vi "bigcryo_Harry-IcT - v1.vi"() -> ()   [LabVIEW 2019]
uses:
  <vilib>/Utility/file.llb/Read From Spreadsheet File (DBL).vi
panel:
  in  "Settle Time (s)":dbl=60.0
  in  "Step/Ramp":bool=TRUE
  in  "T Rate (K/min)":dbl=0.1
  out "Sample Temp - Idle [K]":dbl=1.997
  in  "LakeShore340":refnum<visa-resource-name>="COM7"
  out "dV/dI-I":cluster{dbl[], dbl[]}(graph) caption="XY Graph"
  out "I-V":cluster{dbl[], dbl[]}(graph) caption="XY Graph"
  out "Status":string="Measuring..."
  in  "Stop":bool
  in  "Keithley":refnum<visa-resource-name>="GPIB1::20::INSTR"
  in  "Delay [sec]":dbl=0.002 format="%#_6e"
  in  "Compliance [V] 2":dbl=10.0 format="%#_6f"
  in  "Delta [A]":dbl=1e-05 format="%#_6e"
  in  "Abort Conductance":bool
  in  "Step [A]":dbl=1e-05 format="%#_6e"
  in  "I-Max [A]":dbl=0.002 format="%#_6e"
  in  "Arm Conductance":bool
  in  "Measure":bool
  in  "Directory Output":string="C:\\User Data\\hlb54\\210111_42B\\JJ1\\IcT_test"
  out "T Now":string="2.010"
  in  "Minicryo":bool=TRUE
  in  "Field and rate":dbl[][](array[numeric])
  in  "step":bool=TRUE
  in  "Magnet VISA?":refnum<visa-resource-name>="COM6"
  out "?":refnum<visa-resource-name>="GPIB1::20::INSTR"
  out "Iteration?":i32=401
  out "Path Out":path=path "C:/User Data/hlb54/gigi.dat"
  in  "Start Temp (K)":dbl=2.0 format="%#_7f"
  in  "T Step (K)":dbl=0.01
  out "T Aim":dbl=2.02
  in  "Stop Temp (K)":dbl=2.1
  # "Step"
  # "Ramp"
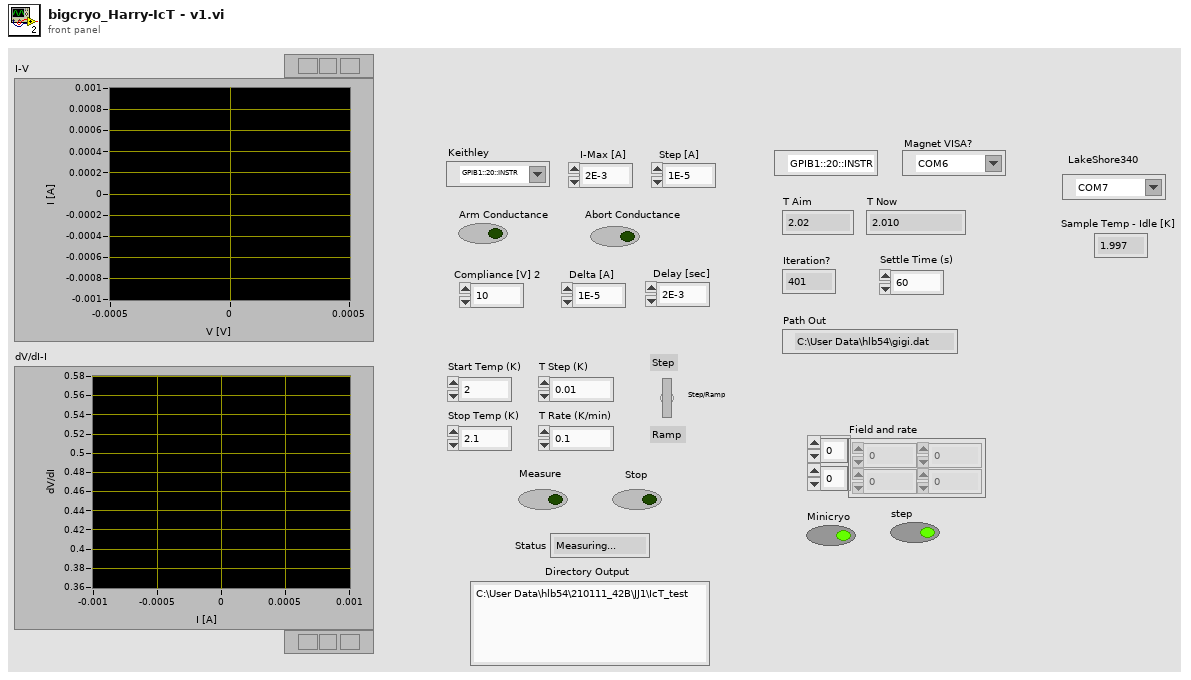
[diagram p1: front panel]
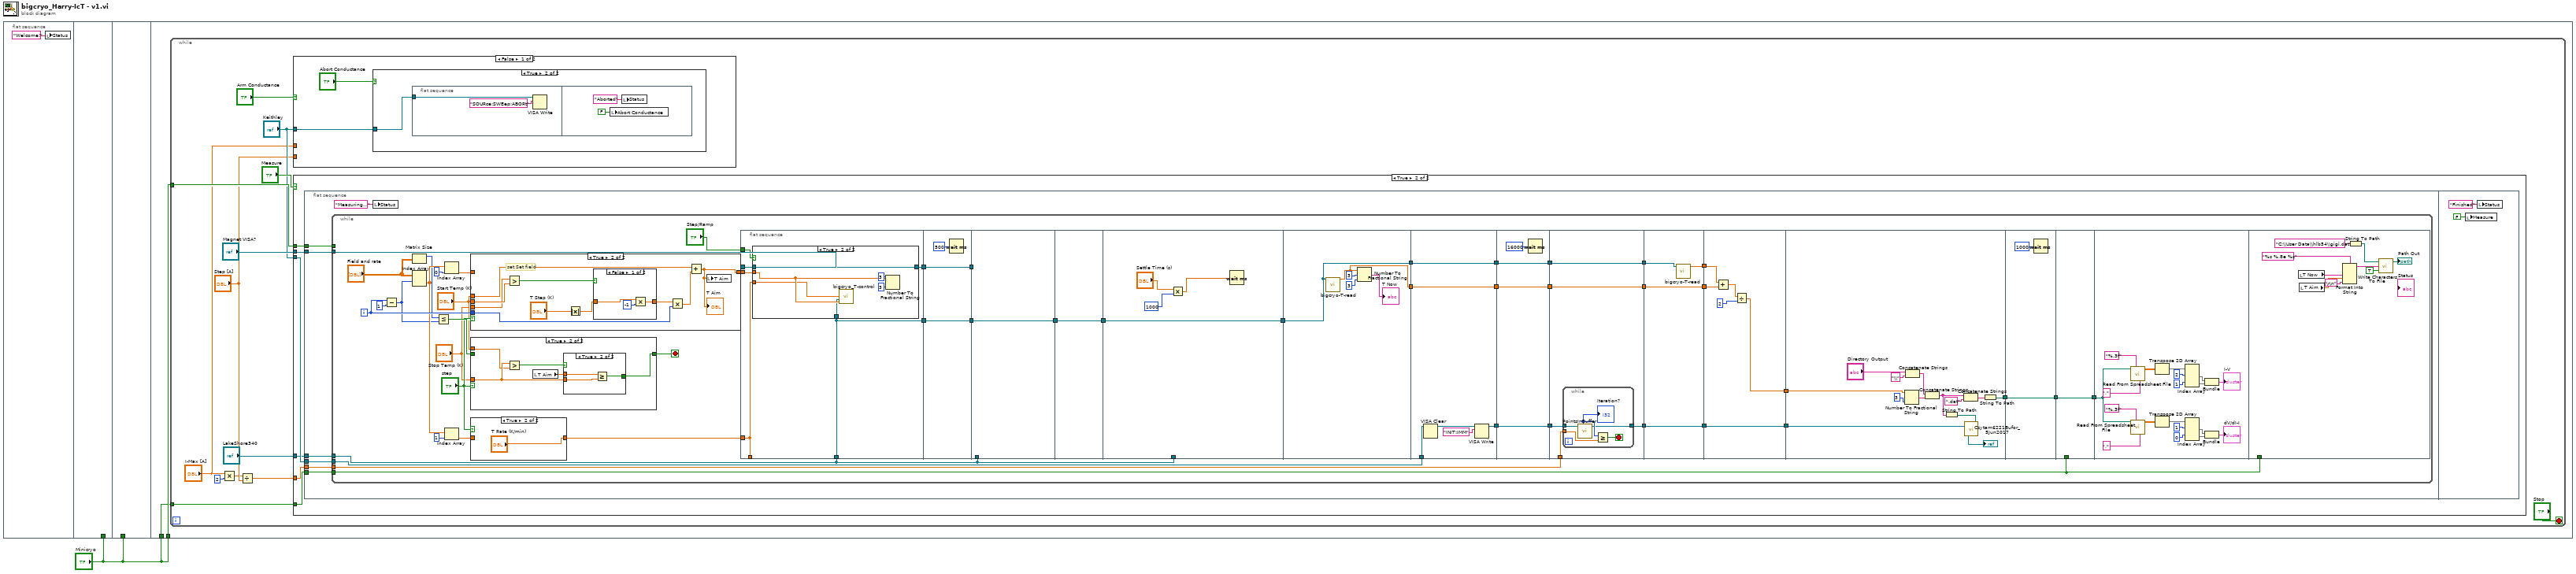
[diagram p0: block diagram]
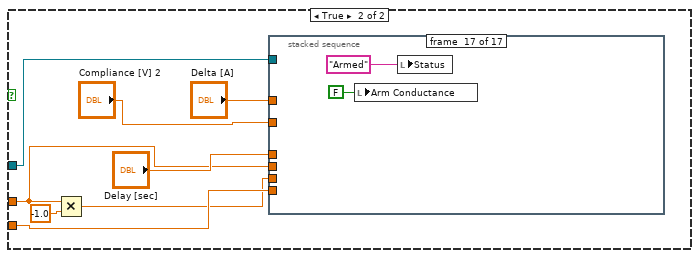
[diagram p3: hidden frame]
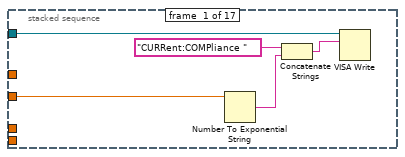
[diagram p4: hidden frame]
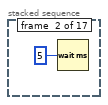
[diagram p5: hidden frame]
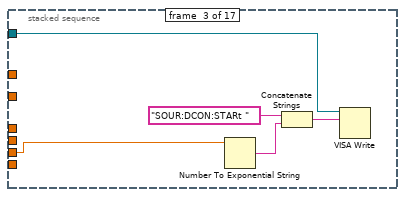
[diagram p6: hidden frame]
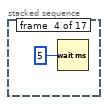
[diagram p7: hidden frame]
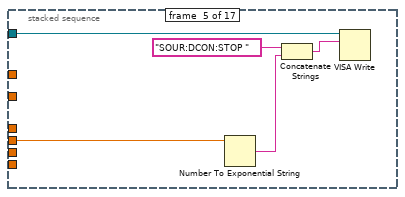
[diagram p8: hidden frame]
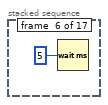
[diagram p9: hidden frame]
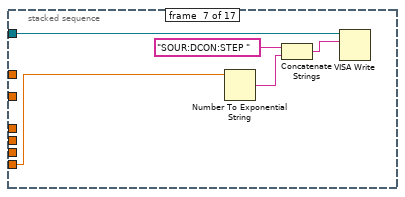
[diagram p10: hidden frame]
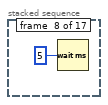
[diagram p11: hidden frame]
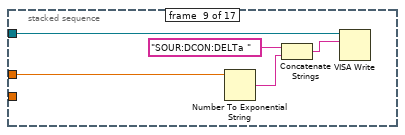
[diagram p12: hidden frame]
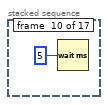
[diagram p13: hidden frame]
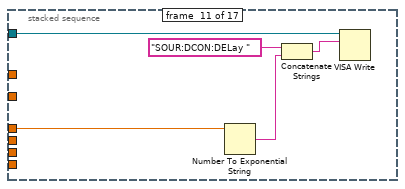
[diagram p14: hidden frame]
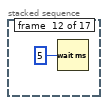
[diagram p15: hidden frame]
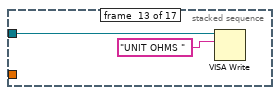
[diagram p16: hidden frame]
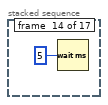
[diagram p17: hidden frame]
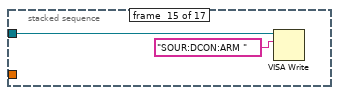
[diagram p18: hidden frame]
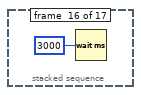
[diagram p19: hidden frame]
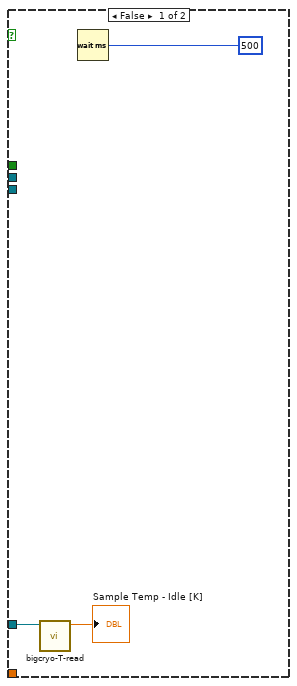
[diagram p20: hidden frame]
diagram:
  n1 = flat-sequence {
    tunnel: "Minicryo" -> [_]
    tunnel: "Minicryo" -> [_]
    tunnel: "Minicryo" -> [w4]
    tunnel: "Minicryo" -> [w3]
    frame #0 {
      n2 = local write "Status"("Welcome!") -> ()
    }
    frame #1 {
    }
    frame #2 {
    }
    frame #3 {
      n3 = while {
        tunnel: w4 -> [w16]
        tunnel: w3 -> [w15]
        stop <- "Stop" stop-if-true
        n4 = Multiply(x="I-Max [A]", y=2) -> (x*y=w6:dbl)
        n5 = Divide(x=w6, y="Step [A]") -> (x/y=w7:dbl)
        n6 = case shown="False" "Arm Conductance" {
          tunnel: "Keithley" -> [w18 w28]
          tunnel: "Step [A]" -> [_ w27]
          tunnel: "I-Max [A]" -> [_ w25]
          frame False {
            n7 = case shown="True" "Abort Conductance" {
              tunnel: w18 -> [_ w20]
              frame False {
              }
              frame True {
                n8 = flat-sequence {
                  tunnel: w20 -> [w21]
                  frame #0 {
                    n9 = VISA Write(VISA resource name=w21, write buffer="SOURce:SWEep:ABORt") -> ()  [unwired: 1 in, 3 out]
                  }
                  frame #1 {
                    n10 = local write "Abort Conductance"(FALSE) -> ()
                    n11 = local write "Status"("Aborted") -> ()
                  }
                }
              }
            }
          }
          frame True {
            n12 = Multiply(x=w25, y=-1.0) -> (x*y=w26:dbl)
            n13 = stacked-sequence {
              tunnel: w26 -> [_ _ w41 _ _ _ _ _ _ _ _ _ _ _ _ _ _]
              tunnel: "Delay [sec]" -> [_ _ _ _ _ _ _ _ _ _ w64 _ _ _ _ _ _]
              tunnel: "Compliance [V] 2" -> [w34 _ _ _ _ _ _ _ _ _ _ _ _ _ _ _ _]
              tunnel: "Delta [A]" -> [_ _ _ _ _ _ _ _ w58 _ _ _ _ _ _ _ _]
              tunnel: w28 -> [w33 _ w39 _ w46 _ w52 _ w57 _ w63 _ w69 _ w72 _ _]
              tunnel: w27 -> [_ _ _ _ _ _ w51 _ _ _ _ _ _ _ _ _ _]
              tunnel: w25 -> [_ _ _ _ w45 _ _ _ _ _ _ _ _ _ _ _ _]
              frame #0 {
                n14 = Number To Exponential String(number=w34) -> (E-format string=w36:string)  [unwired: 3 in]
                n15 = Concatenate Strings("CURRent:COMPliance ", w36) -> (w35:string)
                n16 = VISA Write(VISA resource name=w33, write buffer=w35) -> ()  [unwired: 1 in, 3 out]
              }
              frame #1 {
                n17 = Wait (ms)(milliseconds to wait=5) -> ()  [unwired: 1 out]
              }
              frame #2 {
                n18 = Number To Exponential String(number=w41) -> (E-format string=w42:string)  [unwired: 3 in]
                n19 = Concatenate Strings("SOUR:DCON:STARt ", w42) -> (w40:string)
                n20 = VISA Write(VISA resource name=w39, write buffer=w40) -> ()  [unwired: 1 in, 3 out]
              }
              frame #3 {
                n21 = Wait (ms)(milliseconds to wait=5) -> ()  [unwired: 1 out]
              }
              frame #4 {
                n22 = Number To Exponential String(number=w45) -> (E-format string=w48:string)  [unwired: 3 in]
                n23 = Concatenate Strings("SOUR:DCON:STOP ", w48) -> (w47:string)
                n24 = VISA Write(VISA resource name=w46, write buffer=w47) -> ()  [unwired: 1 in, 3 out]
              }
              frame #5 {
                n25 = Wait (ms)(milliseconds to wait=5) -> ()  [unwired: 1 out]
              }
              frame #6 {
                n26 = Number To Exponential String(number=w51) -> (E-format string=w54:string)  [unwired: 3 in]
                n27 = Concatenate Strings("SOUR:DCON:STEP ", w54) -> (w53:string)
                n28 = VISA Write(VISA resource name=w52, write buffer=w53) -> ()  [unwired: 1 in, 3 out]
              }
              frame #7 {
                n29 = Wait (ms)(milliseconds to wait=5) -> ()  [unwired: 1 out]
              }
              frame #8 {
                n30 = Number To Exponential String(number=w58) -> (E-format string=w60:string)  [unwired: 3 in]
                n31 = Concatenate Strings("SOUR:DCON:DELTa ", w60) -> (w59:string)
                n32 = VISA Write(VISA resource name=w57, write buffer=w59) -> ()  [unwired: 1 in, 3 out]
              }
              frame #9 {
                n33 = Wait (ms)(milliseconds to wait=5) -> ()  [unwired: 1 out]
              }
              frame #10 {
                n34 = Number To Exponential String(number=w64) -> (E-format string=w66:string)  [unwired: 3 in]
                n35 = Concatenate Strings("SOUR:DCON:DELay ", w66) -> (w65:string)
                n36 = VISA Write(VISA resource name=w63, write buffer=w65) -> ()  [unwired: 1 in, 3 out]
              }
              frame #11 {
                n37 = Wait (ms)(milliseconds to wait=5) -> ()  [unwired: 1 out]
              }
              frame #12 {
                n38 = VISA Write(VISA resource name=w69, write buffer="UNIT OHMS ") -> ()  [unwired: 1 in, 3 out]
              }
              frame #13 {
                n39 = Wait (ms)(milliseconds to wait=5) -> ()  [unwired: 1 out]
              }
              frame #14 {
                n40 = VISA Write(VISA resource name=w72, write buffer="SOUR:DCON:ARM ") -> ()  [unwired: 1 in, 3 out]
              }
              frame #15 {
                n41 = Wait (ms)(milliseconds to wait=3000) -> ()  [unwired: 1 out]
              }
              frame #16 {
                n42 = local write "Arm Conductance"(FALSE) -> ()
                n43 = local write "Status"("Armed") -> ()
              }
            }
          }
        }
        n44 = case shown="True" "Measure" {
          tunnel: "Magnet VISA?" -> [_ w85]
          tunnel: w16 -> [_ w84]
          tunnel: w15 -> [_ w83]
          tunnel: "Keithley" -> [_ w82]
          tunnel: w7 -> [_ w81]
          tunnel: "LakeShore340" -> [w77 w80]
          frame False {
            n45 = call "bigcryo-T-read.vi"("Lakeshore Address"=w77) -> ("Sample Temp [K]"=→"Sample Temp - Idle [K]":dbl)  [unwired: 9 in, 1 out]
            n46 = Wait (ms)(milliseconds to wait=u32 500) -> ()  [unwired: 1 out]
          }
          frame True {
            n47 = flat-sequence {
              tunnel: w85 -> [w92]
              tunnel: w84 -> [w91]
              tunnel: w83 -> [w90]
              tunnel: w82 -> [w89]
              tunnel: w81 -> [w88]
              tunnel: w80 -> [w86]
              frame #0 {
                n48 = while {
                  tunnel: w92 -> [w138]
                  tunnel: w91 -> [_]
                  tunnel: w90 -> [w125]
                  tunnel: w89 -> [w123]
                  tunnel: w88 -> [w122]
                  tunnel: w86 -> [w112]
                  i -> [w135]
                  stop <- w121 stop-if-true
                  n49 = Subtract(x=w135, y=1) -> (x-y=w127:i32)
                  n50 = Matrix Size(0:"Field and rate") -> (1:w128:i32)  [unwired: 1 out]
                  n51 = Index Array(array="Field and rate", index (row)=w127) -> (element=w132:dbl[])  [unwired: 1 in]
                  n52 = Less Or Equal?(x=w128, y=w127) -> (x <= y?=w126:bool)
                  n53 = Index Array(array=w132, index=0) -> (element=w131:dbl)
                  n54 = Index Array(array=w132, index=1) -> (element=w130:dbl)
                  n55 = case shown="True" "step" {
                    tunnel: [w156 w165] -> w141
                    tunnel: w135 -> [_ w164]
                    tunnel: w131 -> [w156 _]
                    tunnel: "Start Temp (K)" -> [_ w163]
                    tunnel: "Start Temp (K)" -> [_ w162]
                    tunnel: "Stop Temp (K)" -> [_ w161]
                    frame False {
                    }
                    frame True {
                      # "set Set field"
                      n56 = Greater?(x=w161, y=w162) -> (0:w157:bool)
                      n57 = Absolute Value(x="T Step (K)") -> (abs(x)=w159:dbl)
                      n58 = case shown="False" w157 {
                        tunnel: [w169 w170] -> w158
                        tunnel: w159 -> [w167 w170]
                        frame False {
                          n59 = Multiply(x=w167, y=-1) -> (x*y=w169:dbl)
                        }
                        frame True {
                        }
                      }
                      n60 = Multiply(x=w158, y=w164) -> (x*y=w166:dbl)
                      n61 = Add(x=w163, y=w166) -> (x+y=w165:dbl)
                      "T Aim" <- w165
                      n62 = local write "T Aim"(w165) -> ()
                    }
                  }
                  n63 = case shown="True" "step" {
                    tunnel: [w142 w147] -> w121
                    tunnel: w126 -> [w142 _]
                    tunnel: "Stop Temp (K)" -> [_ w145]
                    tunnel: "Start Temp (K)" -> [_ w144]
                    frame False {
                    }
                    frame True {
                      n64 = Greater?(x=w145, y=w144) -> (0:w143:bool)
                      n65 = local read "T Aim"() -> (w146:dbl)
                      n66 = case shown="True" w143 {
                        tunnel: [w150 w153] -> w147
                        tunnel: w146 -> [w148 w152]
                        tunnel: w145 -> [w149 w151]
                        frame False {
                          n67 = Less Or Equal?(x=w148, y=w149) -> (x <= y?=w150:bool)
                        }
                        frame True {
                          n68 = Greater Or Equal?(x=w152, y=w151) -> (x >= y?=w153:bool)
                        }
                      }
                    }
                  }
                  n69 = case shown="True" "step" {
                    tunnel: [w154 "T Rate (K/min)"] -> w137
                    tunnel: w130 -> [w154 _]
                    frame False {
                    }
                    frame True {
                    }
                  }
                  n70 = flat-sequence {
                    tunnel: w141 -> [w176]
                    tunnel: w138 -> [w175]
                    tunnel: [w174] -> _
                    tunnel: w137 -> [w174]
                    tunnel: "Step/Ramp" -> [w173]
                    tunnel: [w172] -> w115
                    tunnel: w112 -> [w171]
                    tunnel: [w171] -> w111
                    tunnel: w115 -> [w185]
                    tunnel: [w185] -> w114
                    tunnel: w111 -> [w184]
                    tunnel: [w184] -> w110
                    tunnel: w114 -> [_]
                    tunnel: w112 -> [_]
                    tunnel: w110 -> [w187]
                    tunnel: [w187] -> w109
                    tunnel: w109 -> [w188]
                    tunnel: [w188] -> w108
                    tunnel: w112 -> [_]
                    tunnel: w108 -> [w189]
                    tunnel: [w189] -> w107
                    tunnel: w107 -> [w194]
                    tunnel: [w194] -> w105
                    tunnel: [w193] -> w98
                    tunnel: [w201] -> w139
                    tunnel: w123 -> [w200]
                    tunnel: w105 -> [w199]
                    tunnel: [w199] -> w104
                    tunnel: w98 -> [w198]
                    tunnel: [w198] -> w97
                    tunnel: [w207] -> w140
                    tunnel: w139 -> [w207]
                    tunnel: w104 -> [w205]
                    tunnel: [w205] -> w103
                    tunnel: w97 -> [w204]
                    tunnel: [w204] -> w96
                    tunnel: w140 -> [w212]
                    tunnel: [w211] -> w106
                    tunnel: w122 -> [w210]
                    tunnel: w103 -> [w209]
                    tunnel: [w209] -> w102
                    tunnel: w96 -> [w208]
                    tunnel: [w208] -> w95
                    tunnel: w106 -> [w221]
                    tunnel: [w221] -> w101
                    tunnel: w102 -> [w220]
                    tunnel: [w219] -> w99
                    tunnel: w95 -> [w218]
                    tunnel: [w218] -> w94
                    tunnel: w101 -> [w227]
                    tunnel: [w227] -> w100
                    tunnel: w99 -> [w224]
                    tunnel: w94 -> [w223]
                    tunnel: [w222] -> w93
                    tunnel: w100 -> [w236]
                    tunnel: [w232] -> w116
                    tunnel: w93 -> [w228]
                    tunnel: [w241] -> w117
                    tunnel: w116 -> [w241]
                    tunnel: w125 -> [_]
                    tunnel: [w243] -> w118
                    tunnel: w117 -> [w243]
                    tunnel: w118 -> [w244]
                    tunnel: w125 -> [_]
                    frame #0 {
                      n71 = case shown="True" w173 {
                        tunnel: w176 -> [_ w180]
                        tunnel: w175 -> [w177 w181]
                        tunnel: w174 -> [_ w179]
                        tunnel: [w177 w181] -> w172
                        tunnel: w171 -> [_ w178]
                        frame False {
                        }
                        frame True {
                          n72 = call "bigcryo_T-control.vi"("Rate  [K/min]"=w179, "VISA resource name out"=w178, "Set Sample Temp [K]"=w180) -> ()  [unwired: 13 in]
                          n73 = Number To Fractional String(number=w180, width (-)=i16 3, precision (6)=i16 3) -> ()  [unwired: 1 in, 1 out]
                        }
                      }
                    }
                    frame #1 {
                      n74 = Wait (ms)(milliseconds to wait=u32 500) -> ()  [unwired: 1 out]
                    }
                    frame #2 {
                    }
                    frame #3 {
                    }
                    frame #4 {
                      n75 = Multiply(x="Settle Time (s)", y=1000) -> (x*y=w192:dbl)
                      n76 = Wait (ms)(milliseconds to wait=w192) -> ()  [unwired: 1 out]
                    }
                    frame #5 {
                      n77 = call "bigcryo-T-read.vi"("Lakeshore Address"=w194) -> ("Sample Temp [K]"=w193:dbl)  [unwired: 9 in, 1 out]
                      n78 = Number To Fractional String(number=w193, width (-)=i16 3, precision (6)=i16 3) -> (F-format string=→"T Now":string)  [unwired: 1 in]
                    }
                    frame #6 {
                      n79 = VISA Clear(VISA resource name=w200) -> (VISA resource name out=w203:refnum<visa-resource-name>)  [unwired: 1 in, 1 out]
                      n80 = VISA Write(VISA resource name=w203, write buffer="INIT:IMM") -> (VISA resource name out=w201:refnum<visa-resource-name>)  [unwired: 1 in, 2 out]
                    }
                    frame #7 {
                      n81 = Wait (ms)(milliseconds to wait=16000) -> ()  [unwired: 1 out]
                    }
                    frame #8 {
                      n82 = while {
                        tunnel: w212 -> [w215]
                        tunnel: [w214] -> w211
                        tunnel: w210 -> [w213]
                        stop <- w216 stop-if-true
                        n83 = call "PointsInBuffer.vi"("VISA resource name"=w215) -> (3:w214:refnum<visa-resource-name>, "number"=w217:i32)  [unwired: 9 in]
                        "Iteration?" <- w217
                        n84 = Greater Or Equal?(x=w217, y=w213) -> (x >= y?=w216:bool)
                      }
                    }
                    frame #9 {
                      n85 = call "bigcryo-T-read.vi"("Lakeshore Address"=w220) -> ("Sample Temp [K]"=w219:dbl)  [unwired: 9 in, 1 out]
                    }
                    frame #10 {
                      n86 = Add(x=w224, y=w223) -> (x+y=w225:dbl)
                      n87 = Divide(x=w225, y=2) -> (x/y=w222:dbl)
                    }
                    frame #11 {
                      n88 = Number To Fractional String(number=w228, precision (6)=i16 3) -> (F-format string=w240:string)  [unwired: 2 in]
                      n89 = Concatenate Strings("Directory Output", "\\") -> (w229:string)
                      n90 = Concatenate Strings(w229, w240) -> (w234:string)
                      n91 = String To Path(string=w234) -> (path=w239:path)
                      n92 = Concatenate Strings(w234, ".dat") -> (w233:string)
                      n93 = call "Czytam6221Bufor_5Jun2017.vi"("file path (dialog if empty)"=w239, 3:w236) -> (2:→"?":refnum<visa-resource-name>)  [unwired: 1 in]
                      n94 = String To Path(string=w233) -> (path=w232:path)
                    }
                    frame #12 {
                      n95 = Wait (ms)(milliseconds to wait=u32 1000) -> ()  [unwired: 1 out]
                    }
                    frame #13 {
                    }
                    frame #14 {
                      n96 = call-poly <vilib>:"Read From Spreadsheet File.vi"("delimiter (\\t)"="," ("delimiter (\\t)"), "format (%.3f)"="%.3f", "file path (dialog if empty)"=w244) -> ("all rows"=w257:dbl[][])  [unwired: 4 in, 4 out]
                      n97 = call-poly <vilib>:"Read From Spreadsheet File.vi"("delimiter (\\t)"="," ("delimiter (\\t)"), "format (%.3f)"="%.3f", "file path (dialog if empty)"=w244) -> ("all rows"=w248:dbl[][])  [unwired: 4 in, 4 out]
                      n98 = Transpose 2D Array(2D array=w257) -> (transposed array=w256:dbl[][])
                      n99 = Transpose 2D Array(2D array=w248) -> (transposed array=w247:dbl[][])
                      n100 = Index Array(array=w256, index (row) #1=2 ("index (row)"), index (row) #2=1 ("index (row)")) -> (element #1=w259:dbl[], element #2=w258:dbl[])  [unwired: 2 in]
                      n101 = Index Array(array=w247, index (row) #1=1 ("index (row)"), index (row) #2=0 ("index (row)")) -> (element #1=w250:dbl[], element #2=w249:dbl[])  [unwired: 2 in]
                      n102 = Bundle(w259, w258) -> (→"I-V":cluster{dbl[], dbl[]})  [unwired: 1 in]
                      n103 = Bundle(w250, w249) -> (→"dV/dI-I":cluster{dbl[], dbl[]})  [unwired: 1 in]
                    }
                    frame #15 {
                      n104 = local read "T Now"() -> (w266:string)
                      n105 = local read "T Aim"() -> (w263:dbl)
                      n106 = Format Into String(format string="%s %.8e %s", w266, w263, "\r\n") -> (resulting string=w269:string)  [unwired: 2 in, 1 out]
                      n107 = String To Path(string="C:\\User Data\\hlb54\\gigi.dat") -> (path=w264:path)
                      n108 = call <vilib>:"Write Characters To File.vi"("append to file? (new file:F)"=TRUE, "character string"=w269, "file path (dialog if empty)"=w264) -> ("new file path (Not A Path if cancelled)"=→"Path Out":path)  [unwired: 2 out]
                    }
                  }
                }
                n109 = local write "Status"("Measuring...") -> ()
              }
              frame #1 {
                n110 = local write "Measure"(FALSE) -> ()
                n111 = local write "Status"("Finished") -> ()
              }
            }
          }
        }
      }
    }
  }
